vi "OFDM-SIM-Alamouti编码.vi"(0 "调制符号流":cdb[][](array[numeric])) -> (1 "基带信号":cdb[][](array[numeric]), 2 "天线1信号":cdb[][](array[numeric]), 3 "天线2信号":cdb[][](array[numeric]))   [LabVIEW 2018]
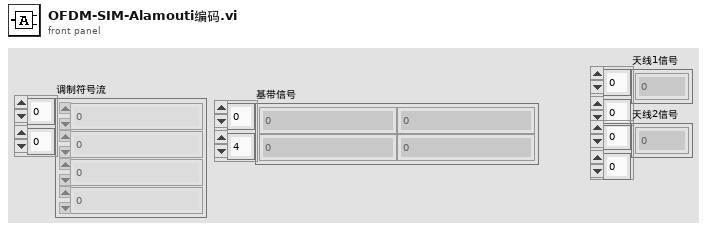
[diagram p1: front panel]
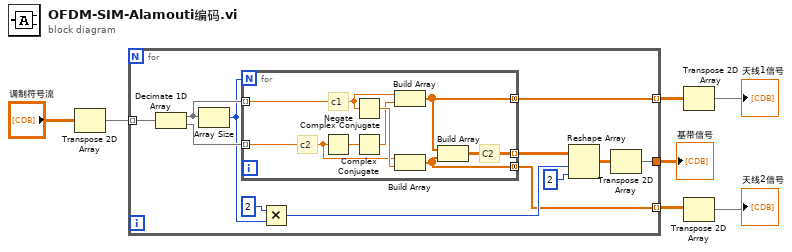
[diagram p0: block diagram]
diagram:
  n1 = Transpose 2D Array(2D array="调制符号流") -> (transposed array=w5:cdb[][])
  n2 = for {
    tunnel: [w15] -> w7
    tunnel: w5 -> [w13] mode=indexing
    tunnel: [w9] -> w2 mode=indexing
    tunnel: [w8] -> w4 mode=indexing
    n3 = Decimate 1D Array(w13) -> (w18:cdb[], w19:cdb[])
    n4 = Array Size(array=w18) -> (size(s)=w12:i32)
    n5 = for {
      N: w12 -> [_]
      tunnel: w19 -> [w21] mode=indexing
      tunnel: w18 -> [w26] mode=indexing
      tunnel: [w24] -> w14 mode=indexing
      tunnel: [w22] -> w8 mode=concatenating
      tunnel: [w20] -> w9 mode=concatenating
      # "C2"
      # "c2"
      # "c1"
      n6 = Negate(x=w21) -> (-x=w27:cdb)
      n7 = Complex Conjugate(1:w26) -> (0:w25:cdb)
      n8 = Complex Conjugate(1:w27) -> (0:w23:cdb)
      n9 = Build Array(w26, w23) -> (w22:cdb[])
      n10 = Build Array(w21, w25) -> (w20:cdb[])
      n11 = Build Array(w22, w20) -> (w24:cdb[][])
    }
    n12 = Multiply(x=2, y=w12) -> (x*y=w11:i32)
    n13 = Reshape Array(w14, w11, 2 ("dimension size")) -> (w17:cdb[][])
    n14 = Transpose 2D Array(2D array=w17) -> (transposed array=w15:cdb[][])
  }
  "基带信号" <- w7
  n15 = Transpose 2D Array(2D array=w4) -> (transposed array=→"天线1信号":cdb[][])
  n16 = Transpose 2D Array(2D array=w2) -> (transposed array=→"天线2信号":cdb[][])
